vi "Select_Focus_Plane.vi"(9 "NewVal":T1 {"Z Steps Size (um)" min=0.0; "Number of Z Steps" min=1; "Frames Accumulations" min=1; "Frames Per Capture" min=1; "Line Accumulations" min=1; "Image Format" items=["64 x 64"=64, "128 x 128"=128, "256 x 256"=256, "512 x 512"=512, "1024 x 1024"=1024, "2048 x 2048"=2048]}, 10 "OldVal":T1 {"Z Steps Size (um)" min=0.0; "Number of Z Steps" min=1; "Frames Accumulations" min=1; "Frames Per Capture" min=1; "Line Accumulations" min=1; "Image Format" items=["64 x 64"=64, "128 x 128"=128, "256 x 256"=256, "512 x 512"=512, "1024 x 1024"=1024, "2048 x 2048"=2048]}, 11 "IntensityGraph in":refnum<vi>) -> ()   [LabVIEW 2016]
uses:
  Type Defs/Image Acquisition Parameters.ctl
panel:
  # "Copyright (C) 2020 Edward S Allgeyer\n\nRedistribution and use in source and binary forms, with or without\nmodification, are permitted provided that the following conditions\nare met:\n\n1. Redistributions of source code must retain the above copyright\n   notice, this list of conditions and the following disclaimer.\n\n2. Redistributions in binary form must reproduce the above copyright\n   notice, this list of conditions and the following disclaimer in\n   the documentation and/or other materials provided with the\n   distribution.\n\n3. Neither the name of the copyright holder nor the names of its\n   contributors may be used to endorse or promote products derived\n   from this software without specific prior written permission.\n\nTHIS SOFTWARE IS PROVIDED BY THE COPYRIGHT HOLDERS AND CONTRIBUTORS\n\"AS IS\" AND ANY EXPRESS OR IMPLIED WARRANTIES, INCLUDING, BUT NOT\nLIMITED TO, THE IMPLIED WARRANTIES OF MERCHANTABILITY AND FITNESS\nFOR A PARTICULAR PURPOSE ARE DISCLAIMED. IN NO EVENT SHALL THE\nCOPYRIGHT HOLDER OR CONTRIBUTORS BE LIABLE FOR ANY DIRECT, INDIRECT,\nINCIDENTAL, SPECIAL, EXEMPLARY, OR CONSEQUENTIAL DAMAGES (INCLUDING,\nBUT NOT LIMITED TO, PROCUREMENT OF SUBSTITUTE GOODS OR SERVICES;\nLOSS OF USE, DATA, OR PROFITS; OR BUSINESS INTERRUPTION) HOWEVER\nCAUSED AND ON ANY THEORY OF LIABILITY, WHETHER IN CONTRACT, STRICT\nLIABILITY, OR TORT (INCLUDING NEGLIGENCE OR OTHERWISE) ARISING IN\nANY WAY OUT OF THE USE OF THIS SOFTWARE, EVEN IF ADVISED OF THE\nPOSSIBILITY OF SUCH DAMAGE."
  # "XY"
  # "Z"
  # "Length"
  # "Height"
  # "XY"
  # "Z"
  # "Length"
  # "Height"
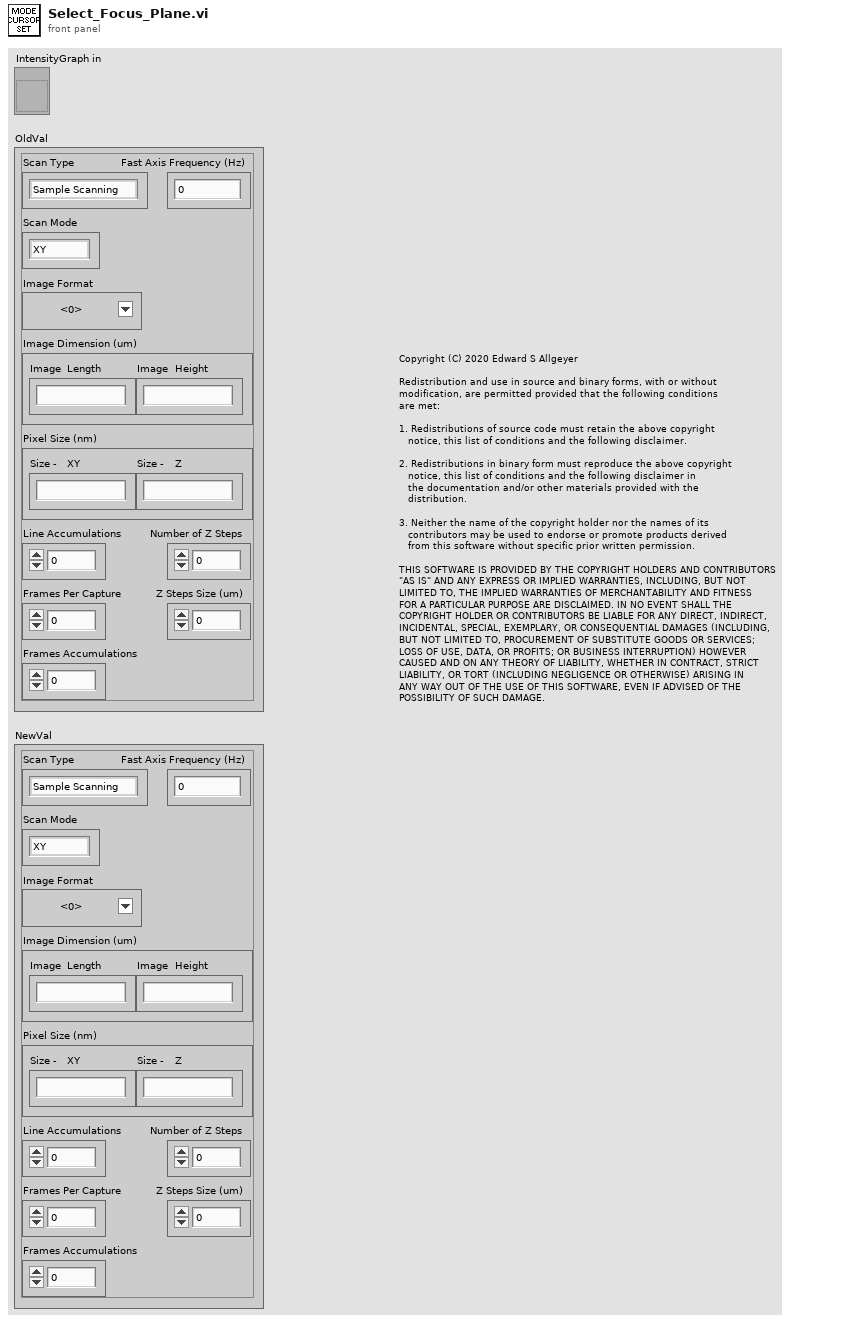
[diagram p1: front panel]
types:
  T1 = typedef "Image Acquisition Parameters.ctl" = cluster{"Scan Type":enum16{"Sample Scanning", "Beam Scanning"}, "Scan Mode":enum16{"XY", "XZ", "YZ", "XYZ"}, "Fast Axis Frequency (Hz)":dbl, "Image Format":u16, "Line Accumulations":u16, "Frames Per Capture":u16, "Frames Accumulations":u16, "Image Dimension (um)":dbl[], "Number of Z Steps":u8, "Z Steps Size (um)":dbl, "Pixel Size (nm)":dbl[]}
  T2 = typedef "Scan Parameters.ctl" = cluster{"Fast_Ax_Amp_V":dbl, "Fast_Ax_Off_V":dbl, "Slow_Ax_Amp_V":dbl, "Slow_Ax_Off_V ":dbl, "Slow_Ax_Max_V_VperS":dbl, "Slow_Ax1_Del25ns":i32, "Slow_Ax2_Del25ns":i32, "Stage_X_Off_V":dbl, "Stage_Y_Off_V":dbl, "Stage_Z_Off_V":dbl, "Galvo1_Off_V":dbl, "Galvo2_Off_V":dbl, "Last_Scan_Mode":enum16{"XY", "XZ", "YZ", "XYZ"}, "Current_Scan_Mode":enum16{"XY", "XZ", "YZ", "XYZ"}, "Fly_Back_Lines":u16, "Linear_Ramp_End":u32, "Z_Step_I16":i16, "Z_Start_I16":i16, "Laser_States _U32":u32, "590_Voltage_I16":i16, "775_AOM_Volt_I16":i16, "Blanking OFF":bool, "Unused_Axis_I16":i16}
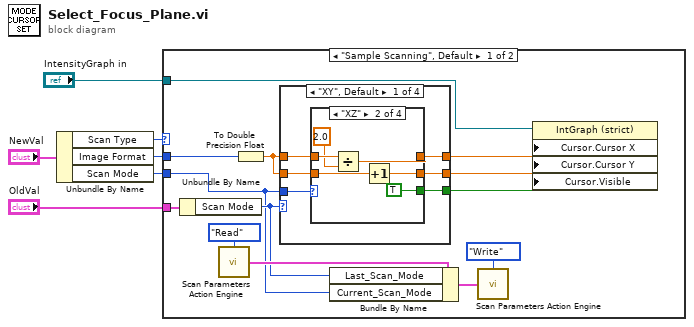
[diagram p0: block diagram]
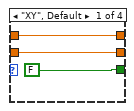
[diagram p2: hidden frame]
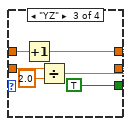
[diagram p3: hidden frame]
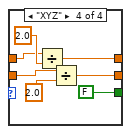
[diagram p4: hidden frame]
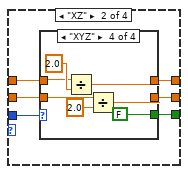
[diagram p5: hidden frame]
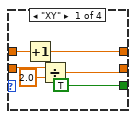
[diagram p6: hidden frame]
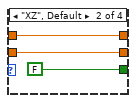
[diagram p7: hidden frame]
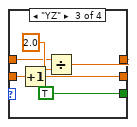
[diagram p8: hidden frame]
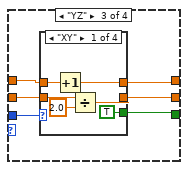
[diagram p9: hidden frame]
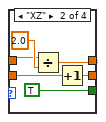
[diagram p10: hidden frame]
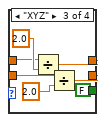
[diagram p11: hidden frame]
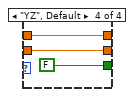
[diagram p12: hidden frame]
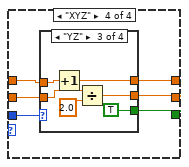
[diagram p13: hidden frame]
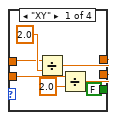
[diagram p14: hidden frame]
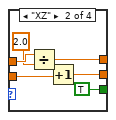
[diagram p15: hidden frame]
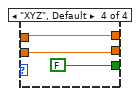
[diagram p16: hidden frame]
diagram:
  n1 = Unbundle By Name("NewVal") -> ("Scan Type"=w6:enum16{"Sample Scanning", "Beam Scanning"}, "Image Format"=w2:u16, "Scan Mode"=w4:enum16{"XY", "XZ", "YZ", "XYZ"})
  n2 = case shown="\"Sample Scanning\", Default" w6 {
    tunnel: w2 -> [w19 _]
    tunnel: "OldVal" -> [w18 _]
    tunnel: w4 -> [w11 _]
    tunnel: "IntensityGraph in" -> [w7 _]
    frame "Sample Scanning", Default {
      n3 = Unbundle By Name(w18) -> ("Scan Mode"=w12:enum16{"XY", "XZ", "YZ", "XYZ"})
      n4 = call "Scan Parameters Action Engine.vi"("Action"=enum16{"Read", "Write"}."Read") -> ("Scan Parameters OUT"=w14:T2)  [unwired: 14 in]
      n5 = To Double Precision Float(number=w19) -> (double precision float=w8:dbl)
      n6 = case shown="\"XY\", Default" w12 {
        tunnel: w8 -> [w24 w52 w80 w108]
        tunnel: w8 -> [w23 w51 w79 w107]
        tunnel: w11 -> [w25 w53 w81 w109]
        tunnel: [w22 w50 w78 w106] -> w17
        tunnel: [w21 w49 w77 w105] -> w16
        tunnel: [w20 w48 w76 w104] -> w15
        frame "XY", Default {
          n7 = case shown="\"XZ\"" w25 {
            tunnel: w24 -> [w27 w34 w39 w41]
            tunnel: w23 -> [w28 w31 w38 w45]
            tunnel: [w27 w30 w36 w42] -> w22
            tunnel: [w28 w29 w35 w46] -> w21
            tunnel: [FALSE ("Cursor.Visible") TRUE ("Cursor.Visible") TRUE ("Cursor.Visible") FALSE ("Cursor.Visible")] -> w20
            frame "XY", Default {
            }
            frame "XZ" {
              n8 = Divide(x=w34, y=2.0) -> (x/y=w29:dbl)
              n9 = Increment(x=w31) -> (x+1=w30:dbl)
            }
            frame "YZ" {
              n10 = Increment(x=w39) -> (x+1=w35:dbl)
              n11 = Divide(x=w38, y=2.0) -> (x/y=w36:dbl)
            }
            frame "XYZ" {
              n12 = Divide(x=w41, y=2.0) -> (x/y=w42:dbl)
              n13 = Divide(x=w45, y=2.0) -> (x/y=w46:dbl)
            }
          }
        }
        frame "XZ" {
          n14 = case shown="\"XYZ\"" w53 {
            tunnel: w52 -> [w55 w62 w66 w69]
            tunnel: w51 -> [w57 w61 w64 w73]
            tunnel: [w54 w62 w63 w70] -> w50
            tunnel: [w56 w61 w65 w74] -> w49
            tunnel: [TRUE ("Cursor.Visible") FALSE ("Cursor.Visible") TRUE ("Cursor.Visible") FALSE ("Cursor.Visible")] -> w48
            frame "XY" {
              n15 = Increment(x=w55) -> (x+1=w54:dbl)
              n16 = Divide(x=w57, y=2.0) -> (x/y=w56:dbl)
            }
            frame "XZ", Default {
            }
            frame "YZ" {
              n17 = Increment(x=w64) -> (x+1=w65:dbl)
              n18 = Divide(x=w66, y=2.0) -> (x/y=w63:dbl)
            }
            frame "XYZ" {
              n19 = Divide(x=w69, y=2.0) -> (x/y=w70:dbl)
              n20 = Divide(x=w73, y=2.0) -> (x/y=w74:dbl)
            }
          }
        }
        frame "YZ" {
          n21 = case shown="\"XY\"" w81 {
            tunnel: w80 -> [w83 w91 w94 w102]
            tunnel: w79 -> [w85 w89 w98 w103]
            tunnel: [w82 w88 w95 w102] -> w78
            tunnel: [w84 w90 w99 w103] -> w77
            tunnel: [TRUE ("Cursor.Visible") TRUE ("Cursor.Visible") FALSE ("Cursor.Visible") FALSE ("Cursor.Visible")] -> w76
            frame "XY" {
              n22 = Increment(x=w83) -> (x+1=w82:dbl)
              n23 = Divide(x=w85, y=2.0) -> (x/y=w84:dbl)
            }
            frame "XZ" {
              n24 = Divide(x=w91, y=2.0) -> (x/y=w88:dbl)
              n25 = Increment(x=w89) -> (x+1=w90:dbl)
            }
            frame "XYZ" {
              n26 = Divide(x=w94, y=2.0) -> (x/y=w95:dbl)
              n27 = Divide(x=w98, y=2.0) -> (x/y=w99:dbl)
            }
            frame "YZ", Default {
            }
          }
        }
        frame "XYZ" {
          n28 = case shown="\"YZ\"" w109 {
            tunnel: w108 -> [w110 w122 w127 w130]
            tunnel: w107 -> [w114 w117 w124 w131]
            tunnel: [w111 w121 w126 w130] -> w106
            tunnel: [w115 w118 w125 w131] -> w105
            tunnel: [FALSE ("Cursor.Visible") TRUE ("Cursor.Visible") TRUE ("Cursor.Visible") FALSE ("Cursor.Visible")] -> w104
            frame "XY" {
              n29 = Divide(x=w110, y=2.0) -> (x/y=w111:dbl)
              n30 = Divide(x=w114, y=2.0) -> (x/y=w115:dbl)
            }
            frame "XZ" {
              n31 = Divide(x=w122, y=2.0) -> (x/y=w121:dbl)
              n32 = Increment(x=w117) -> (x+1=w118:dbl)
            }
            frame "YZ" {
              n33 = Increment(x=w127) -> (x+1=w126:dbl)
              n34 = Divide(x=w124, y=2.0) -> (x/y=w125:dbl)
            }
            frame "XYZ", Default {
            }
          }
        }
      }
      n35 = Bundle By Name(cluster=w14, "Last_Scan_Mode"=w12, "Current_Scan_Mode"=w11) -> (w9:T2)
      n36 = call "Scan Parameters Action Engine.vi"("Action"=enum16{"Read", "Write"}."Write", "Scan Parameters IN"=w9) -> ()  [unwired: 13 in, 1 out]
      n37 = property on="Property Node" class="IntGraph (strict)"(reference=w7, "Cursor.Cursor X"=w17, "Cursor.Cursor Y"=w16, "Cursor.Visible"=w15) -> ()  [unwired: 1 in, 2 out]
    }
    frame "Beam Scanning" {
    }
  }
